vi "przesuwanie wykresu.vi"() -> ()   [LabVIEW 2013]
uses:
  <vilib>/measure/NI_MABase.lvlib
panel:
  out "t max":dbl
  out "t min":dbl
  out "X Scale.Range:Maximum":dbl
  out "X Scale.Range:Minimum":dbl
  in  "stop":bool
  out "Waveform Graph":waveform(dbl)(graph)
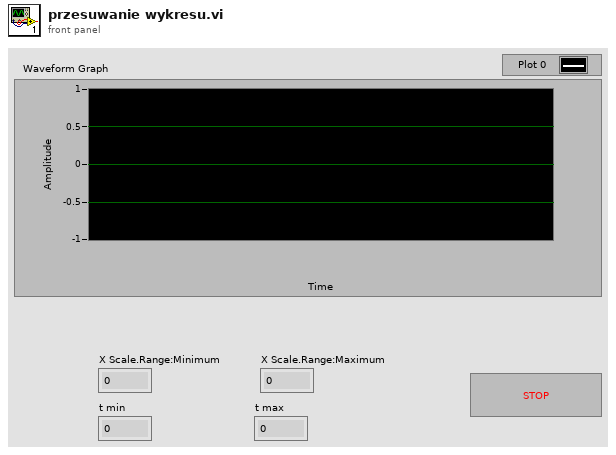
[diagram p1: front panel]
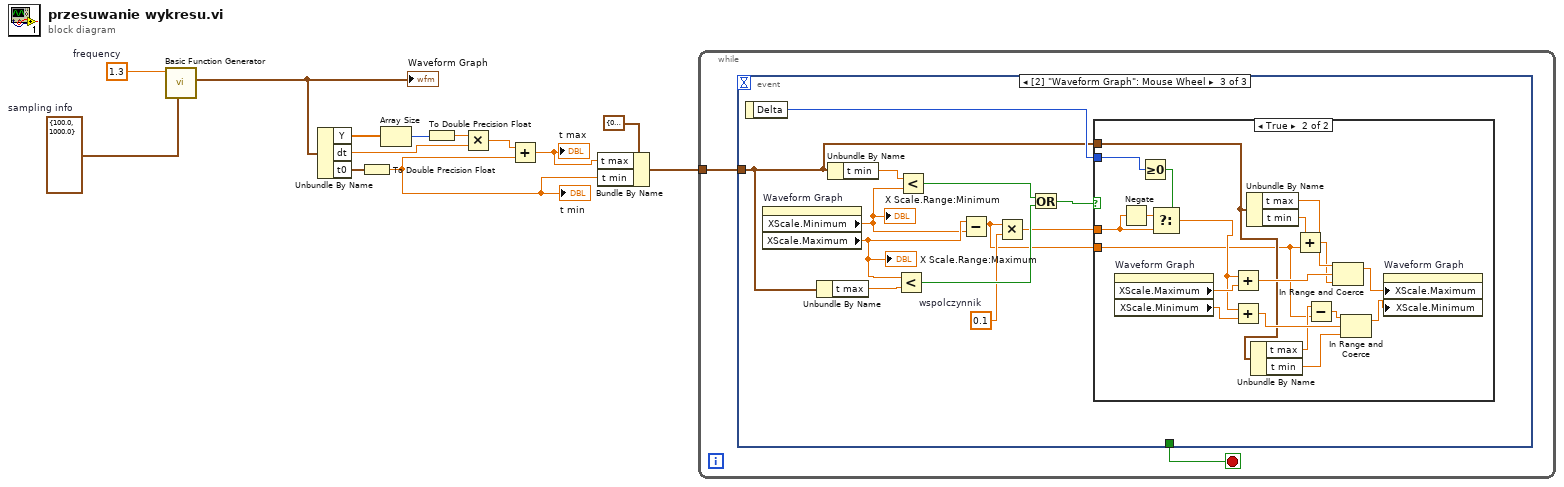
[diagram p0: block diagram]
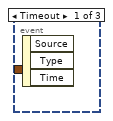
[diagram p2: hidden frame]
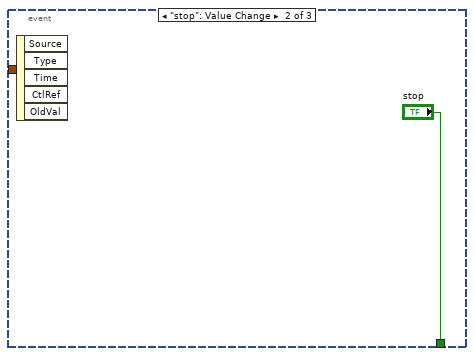
[diagram p3: hidden frame]
diagram:
  w12 = 1.3  # frequency
  w13 = cluster{"Fs":dbl, "#s":dbl} {"Fs"=100.0, "#s"=1000.0}  # sampling info
  n1 = call <vilib>:"Basic Function Generator.vi"("sampling info"=w13, "frequency"=w12) -> ("signal out"=w11:waveform(dbl))  [unwired: 7 in, 2 out]
  "Waveform Graph" <- w11
  n2 = Unbundle By Name(w11) -> ("Y"=w9:dbl[], "dt"=w6:dbl, "t0"=w10:timestamp)
  n3 = To Double Precision Float(number=w10) -> (double precision float=w2:dbl)
  "t min" <- w2
  n4 = Array Size(array=w9) -> (size(s)=w8:i32)
  n5 = To Double Precision Float(number=w8) -> (double precision float=w7:dbl)
  n6 = Multiply(x=w7, y=w6) -> (x*y=w5:dbl)
  n7 = Add(x=w5, y=w2) -> (x+y=w3:dbl)
  "t max" <- w3
  n8 = Bundle By Name(cluster=cluster{"t min":dbl, "t max":dbl} {"t min"=0.0, "t max"=10.0}, "t max"=w3, "t min"=w2) -> (w1:cluster{"t min":dbl, "t max":dbl})
  n9 = while {
    tunnel: w1 -> [w14]
    stop <- w15 stop-if-true
    n10 = event shown="[2] \"Waveform Graph\": Mouse Wheel" {
      selector: _ -> [_ _ _]
      dyn-events: _ -> [_ _ _]
      timeout: _ -> [_ _ _]
      tunnel: [_ "stop" _] -> w15
      tunnel: w14 -> [_ _ w18]
      event Timeout {
        n11 = event-data() -> ()  [unwired: 1 in, 3 out]
      }
      event "stop": Value Change {
        n12 = event-data() -> ()  [unwired: 1 in, 5 out]
      }
      event "Waveform Graph": Mouse Wheel {
        w21 = 0.1  # wspolczynnik
        n13 = event-data() -> ("Delta"=w19:i32)  [unwired: 1 in]
        n14 = property on="Waveform Graph" class="WFGraph (strict)"() -> ("XScale.Minimum"=w23:dbl, "XScale.Maximum"=w24:dbl)  [unwired: 2 in, 2 out]
        "X Scale.Range:Minimum" <- w23
        "X Scale.Range:Maximum" <- w24
        n15 = Unbundle By Name(w18) -> ("t max"=w26:dbl)
        n16 = Unbundle By Name(w18) -> ("t min"=w28:dbl)
        n17 = Less?(x=w24, y=w26) -> (x < y?=w25:bool)
        n18 = Less?(x=w28, y=w23) -> (x < y?=w27:bool)
        n19 = Subtract(x=w24, y=w23) -> (x-y=w17:dbl)
        n20 = Multiply(x=w17, y=w21) -> (x*y=w20:dbl)
        n21 = Or(x=w27, y=w25) -> (x .or. y?=w22:bool)
        n22 = case shown="True" w22 {
          tunnel: w20 -> [_ w32]
          tunnel: w19 -> [_ w45]
          tunnel: w18 -> [_ w35]
          tunnel: w17 -> [_ w29]
          frame False {
          }
          frame True {
            n23 = property on="Waveform Graph" class="WFGraph (strict)"() -> ("XScale.Maximum"=w47:dbl, "XScale.Minimum"=w46:dbl)  [unwired: 2 in, 2 out]
            n24 = Negate(x=w32) -> (-x=w42:dbl)
            n25 = Greater Or Equal To 0?(x=w45) -> (x >= 0?=w44:bool)
            n26 = Select(t=w42, s=w44, f=w32) -> (s? t:f=w43:dbl)
            n27 = Add(x=w43, y=w47) -> (x+y=w41:dbl)
            n28 = Add(x=w43, y=w46) -> (x+y=w36:dbl)
            n29 = Unbundle By Name(w35) -> ("t max"=w40:dbl, "t min"=w39:dbl)
            n30 = Unbundle By Name(w35) -> ("t max"=w33:dbl, "t min"=w34:dbl)
            n31 = Add(x=w39, y=w29) -> (x+y=w38:dbl)
            n32 = Subtract(x=w33, y=w29) -> (x-y=w31:dbl)
            n33 = In Range and Coerce(upper limit=w40, x=w41, lower limit=w38) -> (coerced(x)=w37:dbl)  [unwired: 1 out]
            n34 = In Range and Coerce(upper limit=w31, x=w36, lower limit=w34) -> (coerced(x)=w30:dbl)  [unwired: 1 out]
            n35 = property on="Waveform Graph" class="WFGraph (strict)"("XScale.Maximum"=w37, "XScale.Minimum"=w30) -> ()  [unwired: 2 in, 2 out]
          }
        }
      }
    }
  }
